vi "Handle Error.vi"(8 "error in (no error)":errorcluster, 11 "Template in":refnum<class "Template.lvclass">) -> (0 "error out":errorcluster, 2 "stop actor?":bool=TRUE, 3 "Template out":refnum<class "Template.lvclass">)   [LabVIEW 2020, in "Template.lvlib" / "Template.lvclass"]
doc: "(<B>Filename</B>: Actor Framework.lvlib:Actor.lvclass:Handle Error.vi)\n\nDefines how the actor handles an error that occurred while processing a message. By default, this method does nothing except stop the actor."
uses:
  Template.lvclass
  <vilib>/ActorFramework/Actor/Actor.lvclass
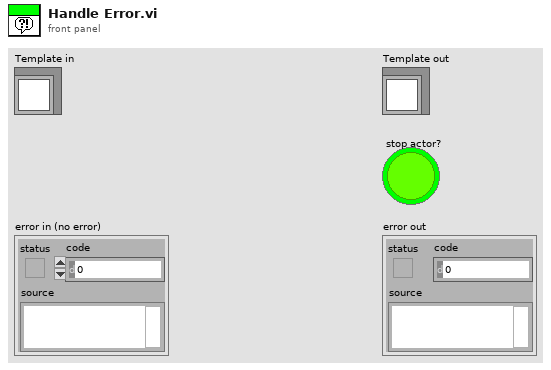
[diagram p1: front panel]
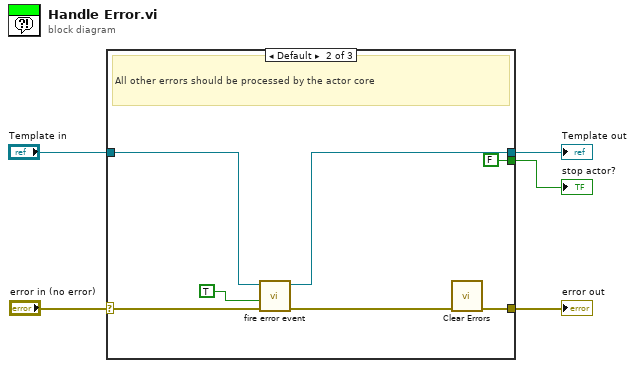
[diagram p0: block diagram]
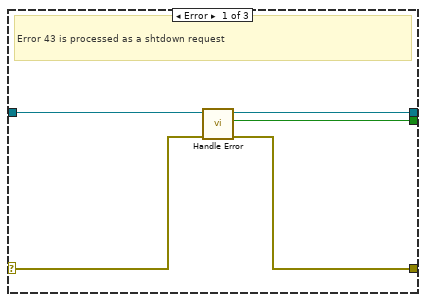
[diagram p2: hidden frame]
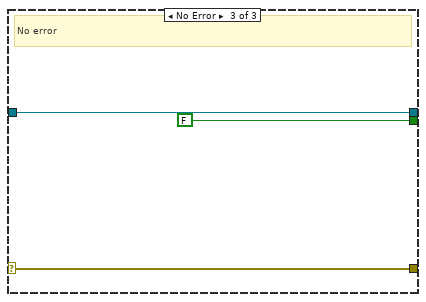
[diagram p3: hidden frame]
diagram:
  n1 = case shown="Default" "error in (no error)" {
    selector: "error in (no error)" -> [w7 w12 w18]
    tunnel: [w10 w14 w18] -> w5
    tunnel: [w9 FALSE ("stop actor?") FALSE ("stop actor?")] -> w4
    tunnel: [w8 w16 w20] -> w3
    tunnel: "Template in" -> [w6 w13 w20]
    frame Error {
      # "Error 43 is processed as a shtdown request"
      n2 = call-parent "Handle Error.vi"("error in (no error)"=w7, "Actor in"=w6) -> ("error out"=w10:errorcluster, "stop actor?"=w9:bool, "Actor out"=w8:refnum<class "Template.lvclass">)  [unwired: 7 in]
    }
    frame Default {
      # "All other errors should be processed by the actor core"
      n3 = call "fire error event.vi"("Error to Process"=w12, "Report Error (F)"=TRUE, "Error Source"=w13) -> ("error out"=w15:errorcluster, "Template out"=w16:refnum<class "Template.lvclass">)  [unwired: 7 in]
      n4 = call <vilib>:"Clear Errors.vi"("error in (no error)"=w15) -> ("error out"=w14:errorcluster)  [unwired: 5 in, 1 out]
    }
    frame No Error {
      # "No error"
    }
  }
  "Template out" <- w3
  "error out" <- w5
  "stop actor?" <- w4
